vi "Write NISTFGenModuleID.vi"(8 "error in (no error)":errorcluster, 10 "NISTFGenModuleID":i32, 11 "NISTBus in":refnum<class "NISTBus.lvclass">) -> (0 "error out":errorcluster, 3 "NISTBus out":refnum<class "NISTBus.lvclass">)   [LabVIEW 2014, in "Bus.lvlib" / "NISTBus.lvclass"]
uses:
  Test/Bus/NISTBus.lvclass
  Test/Bus/NISTBus.lvclass/NISTBus.ctl
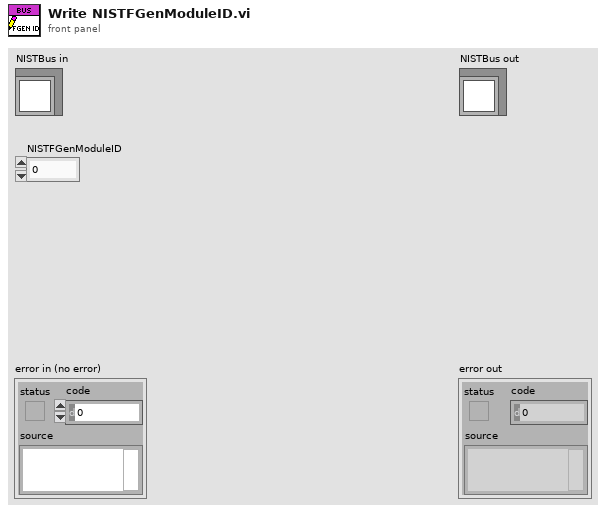
[diagram p1: front panel]
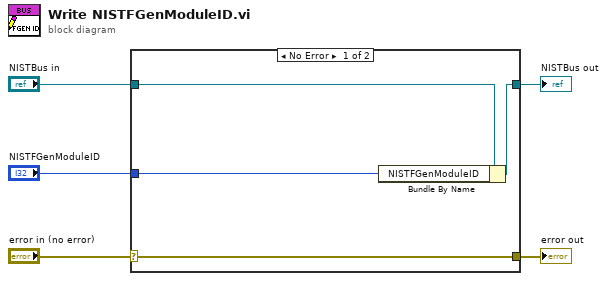
[diagram p0: block diagram]
diagram:
  n1 = case shown="No Error" "error in (no error)" {
    selector: "error in (no error)" -> [w9 w10]
    tunnel: [w9 w10] -> w4
    tunnel: [w7 w11] -> w2
    tunnel: "NISTBus in" -> [w8 w11]
    tunnel: "NISTFGenModuleID" -> [w6 _]
    frame No Error {
      n2 = Bundle By Name(cluster=w8, "NISTFGenModuleID"=w6) -> (w7:refnum<class "NISTBus.lvclass">)
    }
    frame Error {
    }
  }
  "error out" <- w4
  "NISTBus out" <- w2
